vi "voltech360.vi"() -> ()   [LabVIEW 2015]
uses:
  <instrlib>/Voltech PM1000+/Public/Configure/Configure Measurements (Normal).vi
  <vilib>/Utility/file.llb/Write Delimited Spreadsheet (string).vi
  <instrlib>/Voltech PM1000+/Voltech PM1000+.lvlib
panel:
  in  "Minutes per test":dbl
  in  "FOLDER NAME":string
  in  "HOW MANY TEST":i32
  in  "Name of File":string
  in  "VISA resource name 2":refnum<visa-resource-name>
  out "Current Data Point":i32
  in  "stop":bool
  out "VRMS":dbl[](graph)
  in  "Normal Measurements":i32[](listbox)=[0, 1, 2, 3, 4, 5, 6]
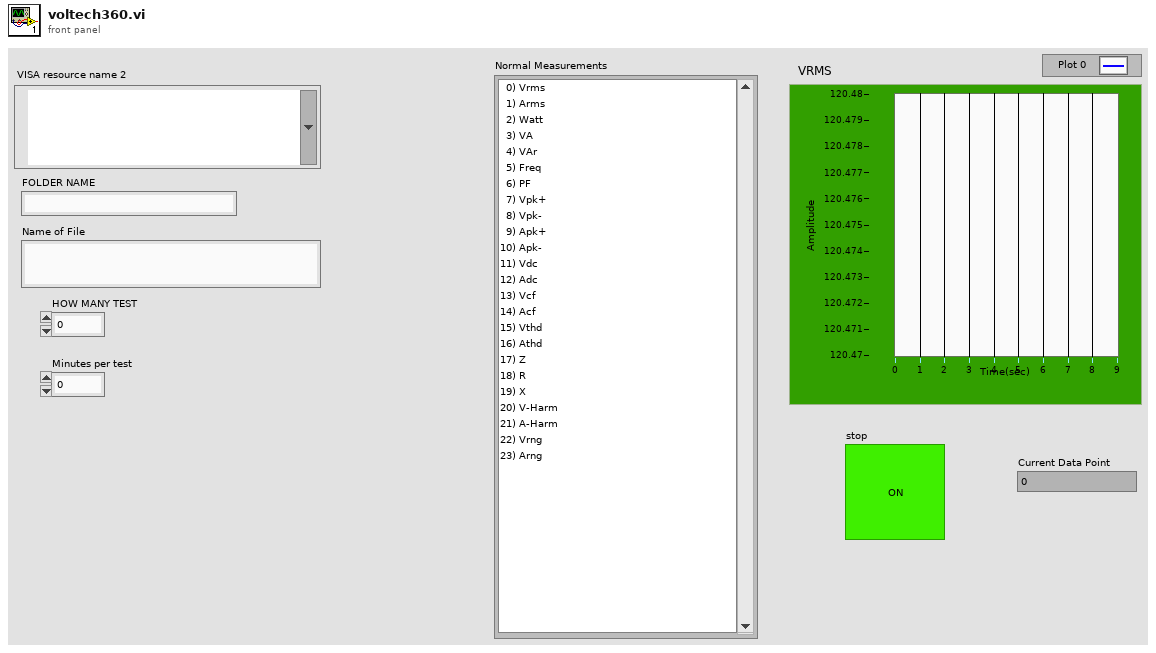
[diagram p1: front panel]
types:
  T1 = enum16{"open", "replace", "create", "open or create", "replace or create", "replace or create with confirmation"}
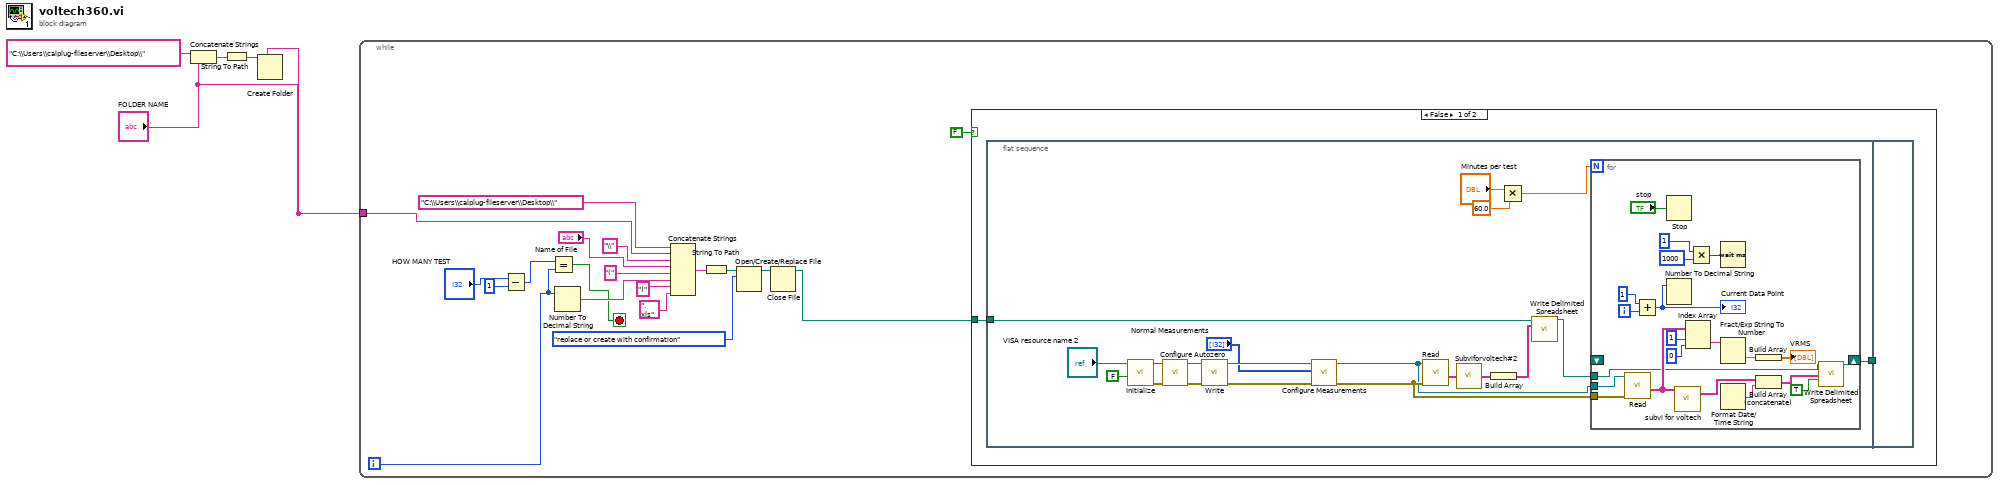
[diagram p0: block diagram]
diagram:
  n1 = Concatenate Strings("C:\\Users\\calplug-fileserver\\Desktop\\" ("string"), "FOLDER NAME") -> (w4:string)
  n2 = String To Path(string=w4) -> (path=w3:path)
  n3 = Create Folder(prompt (Create Folder)="FOLDER NAME", path (use dialog)=w3) -> ()  [unwired: 1 in, 3 out]
  n4 = while {
    tunnel: "FOLDER NAME" -> [w8]
    i -> [w9]
    stop <- w10 stop-if-true
    n5 = Subtract(x="HOW MANY TEST", y=1) -> (x-y=w5:i32)
    n6 = Equal?(x=w5, y=w9) -> (x = y?=w10:bool)
    n7 = Number To Decimal String(number=w9) -> (decimal integer string=w15:string)  [unwired: 1 in]
    n8 = Concatenate Strings("C:\\Users\\calplug-fileserver\\Desktop\\" ("string"), w8, "\\" ("string"), "Name of File", "(" ("string"), w15, ")" ("string"), ".xls" ("string")) -> (w20:string)
    n9 = String To Path(string=w20) -> (path=w21:path)
    n10 = Open/Create/Replace File(file path (use dialog)=w21, operation (0:open)=T1."replace or create with confirmation") -> (refnum out=w19:refnum<file>)  [unwired: 4 in, 2 out]
    n11 = Close File(refnum=w19) -> (path=w11:path)  [unwired: 1 in, 1 out]
    n12 = case shown="False" FALSE {
      tunnel: w11 -> [w25 _]
      frame False {
        n13 = flat-sequence {
          tunnel: w25 -> [w26]
          tunnel: [w41] -> w24
          tunnel: w24 -> [_]
          frame #0 {
            n14 = call <instrlib>:"Initialize.vi"("Reset (True)"=FALSE, "VISA resource name"="VISA resource name 2") -> ("error out"=w43:errorcluster, "VISA resource name out"=w44:refnum<visa-resource-name>)  [unwired: 8 in]
            n15 = call <instrlib>:"Configure Autozero.vi"("error in (no error)"=w43, "VISA resource name"=w44) -> ("error out"=w39:errorcluster, "VISA resource name out"=w40:refnum<visa-resource-name>)  [unwired: 8 in]
            n16 = call <instrlib>:"Write.vi"("error in (no error)"=w39, "VISA resource name"=w40) -> ("error out"=w37:errorcluster, "VISA resource name out"=w38:refnum<visa-resource-name>)  [unwired: 8 in]
            n17 = call-poly <instrlib>:"Configure Measurements.vi"("error in (no error)"=w37, "Normal Measurements"="Normal Measurements", "VISA resource name"=w38) -> ("error out"=w33:errorcluster, "VISA resource name out"=w32:refnum<visa-resource-name>)  [unwired: 7 in]
            n18 = call <instrlib>:"Read.vi"("error in (no error)"=w33, "VISA resource name"=w32) -> ("Measurement Results"=w34:string[][])  [unwired: 7 in, 2 out]
            n19 = call "Subviforvoltech#2.vi"("Measurement Results 2"=w34) -> ("Array"=w36:string[])
            n20 = Build Array(w36) -> (w27:string[][])
            n21 = Multiply(x="Minutes per test", y=60.0) -> (x*y=w31:dbl)
            n22 = call-poly <vilib>:"Write Delimited Spreadsheet.vi"("file path (dialog if empty)"=w26, "2D data"=w27) -> ("new file path (Not A Path if cancelled)"=w28:path)  [unwired: 12 in, 1 out]
            n23 = for {
              N: w31 -> [_]
              tunnel: w28 -> [w48]
              shift-right: [w46] -> w41
              shift-left: _ -> [_]
              tunnel: w32 -> [w60]
              tunnel: w33 -> [w59]
              i -> [w63]
              n24 = call <instrlib>:"Read.vi"("error in (no error)"=w59, "VISA resource name"=w60) -> ("Measurement Results"=w51:string[][])  [unwired: 7 in, 2 out]
              n25 = Add(x=1, y=w63) -> (x+y=w64:i32)
              "Current Data Point" <- w64
              n26 = Stop(stop? (T)="stop") -> ()
              n27 = Number To Decimal String(number=w64) -> ()  [unwired: 1 in, 1 out]
              n28 = call "subvi for voltech.vi"("Measurement Results 2"=w51) -> ("Array"=w61:string[])  [unwired: 6 in]
              n29 = Index Array(array=w51, index (row)=1, index (col)=0 ("disabled index (col)")) -> (element=w54:string)
              n30 = Multiply(x=u32 1 ("Interval of Data Collection (sec)"), y=u32 1000) -> (x*y=w65:u32)
              n31 = Wait (ms)(milliseconds to wait=w65) -> ()  [unwired: 1 out]
              n32 = Fract/Exp String To Number(string=w54) -> (number=w50:dbl)  [unwired: 3 in, 1 out]
              n33 = Format Date/Time String() -> (date/time string=w57:string)  [unwired: 3 in]
              n34 = Build Array(w50) -> (→"VRMS":dbl[])
              n35 = Build Array (concatenate)(w61, w57) -> (w47:string[])
              n36 = call-poly <vilib>:"Write Delimited Spreadsheet.vi"("file path (dialog if empty)"=w48, "1D data"=w47, "append to file? (F)"=TRUE ("append to file? (new file:F)")) -> ("new file path (Not A Path if cancelled)"=w46:path)  [unwired: 11 in, 1 out]
            }
          }
          frame #1 {
          }
        }
      }
      frame True {
      }
    }
  }
